vi "svfa_Window Frequency Response (double).vi"(1 "N (window length)":i32=512, 2 "window":T1(ring), 3 "f(normalized)":dbl format="%.5f") -> (0 "H(f)":cdb format="%.5e")   [LabVIEW 2017]
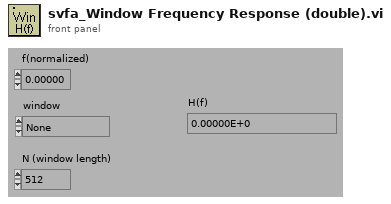
[diagram p1: front panel]
types:
  T1 = enum16{"None ", "Hanning", "Hamming", "Blackman-Harris", "Exact Blackman", "Blackman", "Flat Top", "4 Term B-Harris ", "7 Term B-Harris", "Low Sidelobe"}
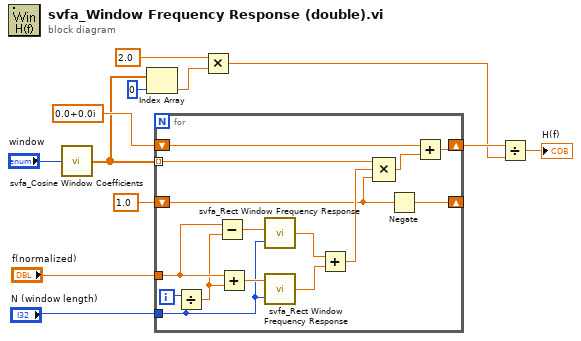
[diagram p0: block diagram]
diagram:
  n1 = call <vilib>:"svfa_Cosine Window Coefficients.vi"("window"="window") -> ("WinCoefficients"=w5:dbl[])
  n2 = Index Array(array=w5, index=0 ("Index")) -> (element=w8:dbl)
  n3 = for {
    tunnel: w5 -> [w24] mode=indexing
    tunnel: "f(normalized)" -> [w21]
    tunnel: "N (window length)" -> [w17]
    shift-right: [w25] -> w11
    shift-left: cdb 0.0+0.0i -> [w26]
    shift-right: [w14] -> _
    shift-left: 1.0 ("y") -> [w13]
    i -> [w27]
    n4 = Divide(x=w27, y=w17) -> (x/y=w20:dbl)
    n5 = Subtract(x=w21, y=w20) -> (x-y=w18:dbl)
    n6 = Add(x=w21, y=w20) -> (x+y=w19:dbl)
    n7 = call <vilib>:"svfa_Rect Window Frequency Response.vi"("N"=w17, "f"=w18) -> ("H(f)"=w16:cdb)
    n8 = call <vilib>:"svfa_Rect Window Frequency Response.vi"("N"=w17, "f"=w19) -> ("H(f)"=w15:cdb)
    n9 = Add(x=w16, y=w15) -> (x+y=w23:cdb)
    n10 = Compound Arithmetic op=MULTIPLY(w24, w23, w13) -> (w22:cdb)
    n11 = Negate(x=w13) -> (-x=w14:dbl)
    n12 = Add(x=w26, y=w22) -> (x+y=w25:cdb)
  }
  n13 = Multiply(x=2.0 ("y"), y=w8) -> (x*y=w7:dbl)
  n14 = Divide(x=w11, y=w7) -> (x/y=→"H(f)":cdb)
